vi "beepalert.vi"(10 "duration (msec)":u32=100, 11 "frequency (Hz)":u32) -> ()   [LabVIEW 2015]
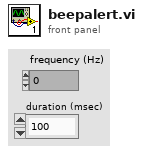
[diagram p1: front panel]
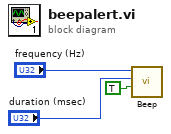
[diagram p0: block diagram]
diagram:
  n1 = call <vilib>:"Beep.vi"("use system alert? (T)"=TRUE, "duration (msec)"="duration (msec)", "frequency (Hz)"="frequency (Hz)") -> ()  [unwired: 9 in]
